vi "GUI_LP.vi"() -> ()   [LabVIEW 2013]
uses:
  Shared/GUI_Template/GUI_master/tcp_new_data_event.ctl
  Shared/GUI_Template/GUI_master/tcp new data cluster.ctl
panel:
  in  "GUIdevice 1":string="SmaractFilter-1"
  in  "Position.Channel 3::1":dbl caption="Position (LP Mode - CH3)" min=0.0 max=75.0 format="%#_6p"
  in  "stop":bool
  in  "insert tag":bool=TRUE
  out "error IO 2":errorcluster
  out "tcp data event":T1
  in  "Camera Stage":dbl(slide) scale=0.0..75.0
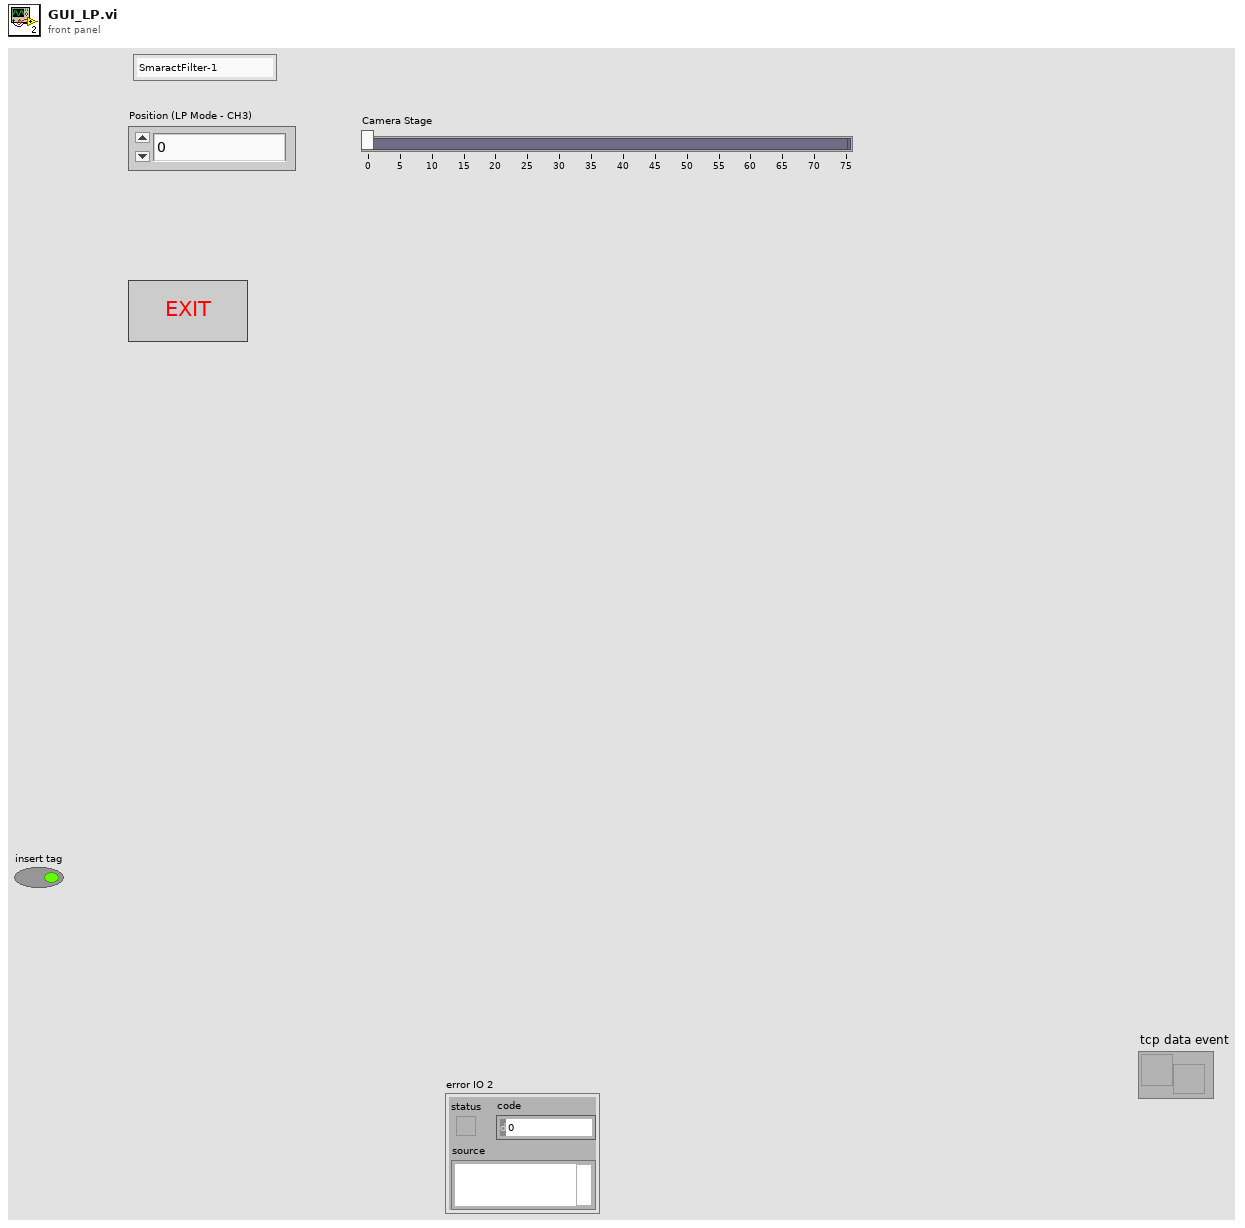
[diagram p1: front panel]
types:
  T1 = typedef "tcp_new_data_event.ctl" = refnum<user-event>
  T2 = typedef "tcp new data cluster.ctl" = cluster{"EventEnum":enum16{"new data", "connection status update"}, "Device name":string}
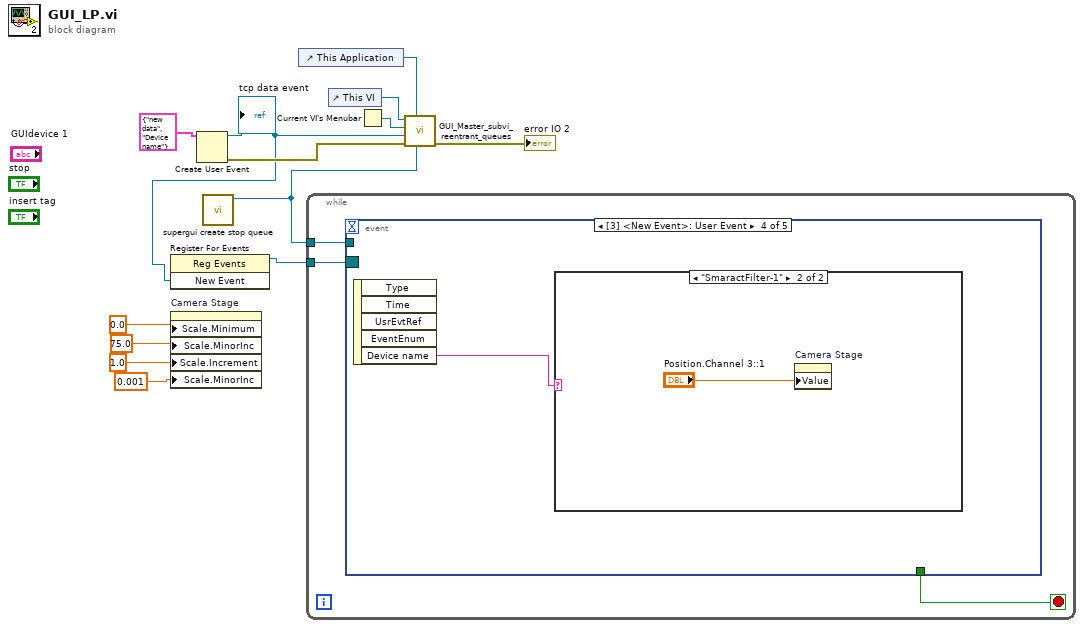
[diagram p0: block diagram]
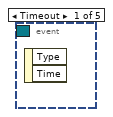
[diagram p2: hidden frame]
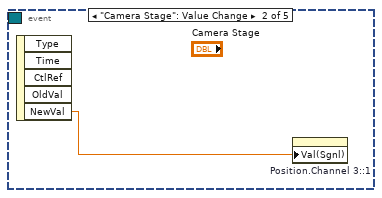
[diagram p3: hidden frame]
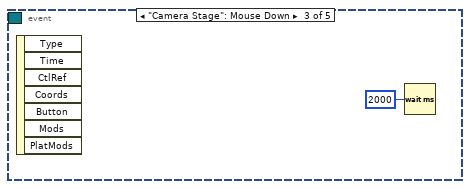
[diagram p4: hidden frame]
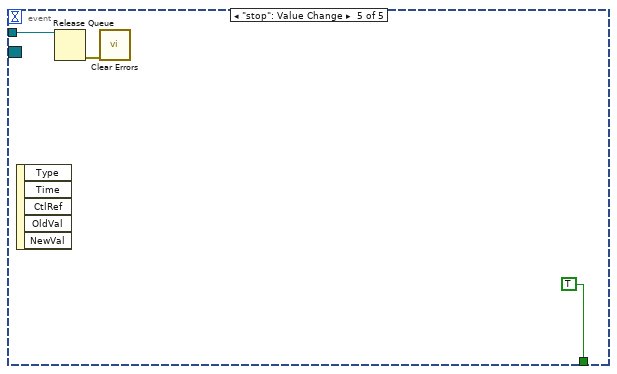
[diagram p6: hidden frame]
diagram:
  n1 = property on="Camera Stage" class="Slide (strict)"("Scale.Minimum"=0.0 ("Doc Min"), "Scale.MinorInc"=75.0 ("Doc Max"), "Scale.Increment"=1.0 ("Increment"), "Scale.MinorInc"=0.001 ("Increment")) -> ()  [unwired: 2 in, 2 out]
  n2 = Create User Event(user event datatype=T2 {"EventEnum"=enum."new data", "Device name"="Device name"} ("New Event")) -> (user event=w6:refnum<user-event>, error out=w12:errorcluster)  [unwired: 1 in]
  "tcp data event" <- w6
  n3 = register-events(w6) -> (reference out=w7:refnum<event-registration>)  [unwired: 2 in, 1 out]
  n4 = call "supergui create stop queue.vi"() -> ("STOP Queue out"=w1:refnum<queue>)  [unwired: 11 in]
  n5 = control-ref of="This Application"() -> (w13:refnum<vi>)
  n6 = while {
    tunnel: w7 -> [w15]
    tunnel: w1 -> [w14]
    stop <- w16 stop-if-true
    n7 = event shown="[3] <New Event>: User Event" {
      selector: w15 -> [_ _ _ _ _]
      dyn-events: _ -> [_ _ _ _ _]
      timeout: _ -> [_ _ _ _ _]
      tunnel: [_ _ _ _ TRUE] -> w16
      tunnel: w14 -> [_ _ _ _ w22]
      event Timeout {
        n8 = event-data() -> ()  [unwired: 1 in, 2 out]
      }
      event "Camera Stage": Value Change {
        n9 = event-data() -> ("NewVal"=w17:dbl)  [unwired: 1 in, 4 out]
        n10 = property on="Position.Channel 3::1" class="DigNum (strict)"("Val(Sgnl)"=w17) -> ()  [unwired: 2 in, 2 out]
      }
      event "Camera Stage": Mouse Down {
        n11 = event-data() -> ()  [unwired: 1 in, 7 out]
        n12 = Wait (ms)(milliseconds to wait=u32 2000) -> ()  [unwired: 1 out]
      }
      event User Event {
        n13 = event-data() -> ("Device name"=w19:string)  [unwired: 1 in, 4 out]
        n14 = case shown="\"SmaractFilter-1\"" w19 {
          frame "False", Default {
          }
          frame "SmaractFilter-1" {
            n15 = property on="Camera Stage" class="Slide (strict)"("Value"="Position.Channel 3::1") -> ()  [unwired: 2 in, 2 out]
          }
        }
      }
      event "stop": Value Change {
        n16 = event-data() -> ()  [unwired: 1 in, 5 out]
        n17 = Release Queue(queue=w22) -> (error out=w21:errorcluster)  [unwired: 2 in, 2 out]
        n18 = call <vilib>:"Clear Errors.vi"("error in (no error)"=w21) -> ()  [unwired: 6 in, 1 out]
      }
    }
  }
  n19 = control-ref of="This VI"() -> (w9:refnum<vi>)
  n20 = Current VI's Menubar() -> (w10:refnum<k9>)
  n21 = call "GUI_Master_subvi_reentrant_queues.vi"("STOP Queue in"=w1, "This Application"=w13, "error in (no error)"=w12, "tcp data event"=w6, "Caller menu reference"=w10, "Caller VI ref"=w9) -> ("error out"=→"error IO 2":errorcluster)  [unwired: 5 in]
